vi "Automatic Assembly DB.vi"() -> ()   [LabVIEW 2021]
uses:
  Classes/Assembly/Assembly Run.lvclass
  Classes/Assembly/Database Entry/Database Entry.lvclass
  <vilib>/Utility/file.llb/Read Delimited Spreadsheet (string).vi
  SubVIs/PUT_region.vi
  SubVIs/component_tray_region.vi
  SubVIs/assembly_tray_region.vi
  Classes/Controller/I-O/I-O.lvclass
  Classes/Controller/Controller.lvclass
panel:
  in  "Abort assembly":bool
  in  "Do old-style single-module data-entry?":bool
  out "Status":string
  out "Stack names":T1
  out "Feet check":bool
  out "Assembly Type":string
  out "Assembly tray region":dbl
  out "Component tray region":dbl
  out "PUT Region":dbl
  # "Click the Run arrow to start.\nFill out pop-up prompts.\nSee Status for more info.\nAnswer ALL prompts until program stops running!"
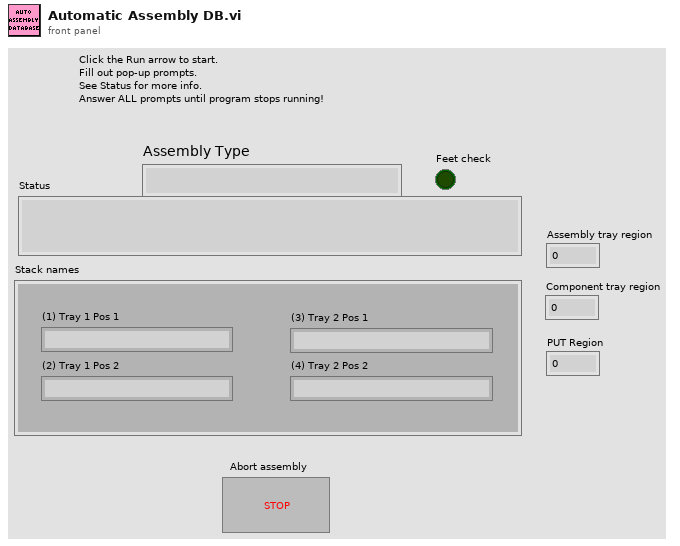
[diagram p1: front panel]
types:
  T1 = cluster{"(1) Tray 1 Pos 1":string, "(2) Tray 1 Pos 2":string, "(3) Tray 2 Pos 1":string, "(4) Tray 2 Pos 2":string}
  T2 = typedef "Controller.lvclass/Controllers.ctl" = cluster{"I-O.lvclass":refnum<class "I-O.lvclass">, "Gantry":refnum<k24>, "Dispenser":refnum<visa-resource-name>}
  T3 = typedef "File Paths.ctl" = cluster{"Glue Pattern Folder":path, "Carrier Tray Folder":path, "Pick Up Tool Fixture Folder":path, "Components Folder":path, "Bellows Tool Offset.txt":path, "Pick Up Tool Offset.txt":path, "Dispense Tip Offset.txt":path, "Log Files":path, "Gantry Assembly Map.txt":path, "Syringe and offset map.txt":path, "Controllers Folder":path, "Local dbase config":path}
  T4 = cluster{"Fixture ID":dbl, "Position":dbl, "Thickness":dbl}[]
  T5 = cluster{"Fixture ID":dbl, "Position":dbl, "Thickness":dbl}[][]
  T6 = cluster{"Fixture ID":dbl, "Position":dbl, "Thickness":dbl}
  T7 = typedef "I-O.lvclass/Pin Map.ctl" = cluster{"Region Valves":i32[], "Extra Valves":dbl[][][], "Tool Primary Valve":i32, "Tool Secondary Valve":i32, "Region Sensors":i32[], "Extra Sensors":dbl[][][], "Tool Primary Sensor":dbl, "Tool Secondary Sensor":dbl, "Compression Sensor":dbl, "5V":i32, "Dispenser Sensor":dbl, "Light Curtain":i32}
  T8 = cluster{"Stack names[0]":string, "Stack names[1]":string, "Stack names[2]":string, "Stack names[3]":string}
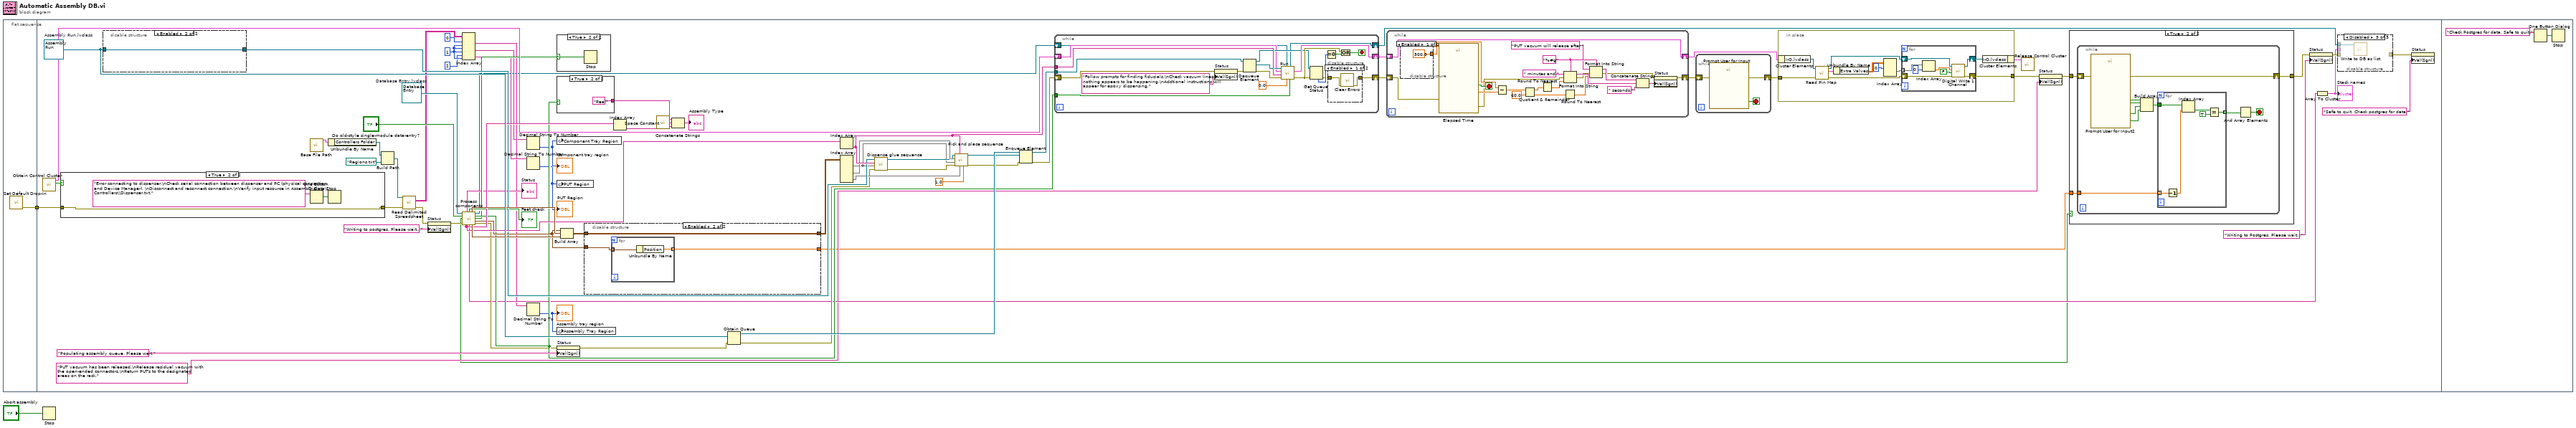
[diagram p0: block diagram]
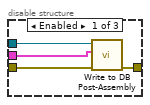
[diagram p3: hidden frame]
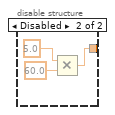
[diagram p5: hidden frame]
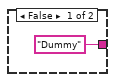
[diagram p7: hidden frame]
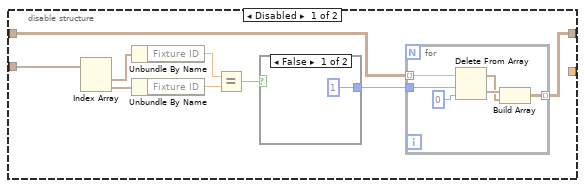
[diagram p9: hidden frame]
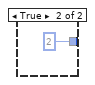
[diagram p10: hidden frame]
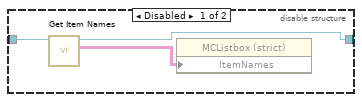
[diagram p11: hidden frame]
diagram:
  n1 = flat-sequence {
    tunnel: [w3] -> w2
    tunnel: w2 -> [w21]
    frame #0 {
      n2 = call "Set Default Drop-In.vi"() -> ("error out"=w3:errorcluster)  [unwired: 11 in]
    }
    frame #1 {
      w26 = 1 ("disabled index (col)")
      w49 = refnum<class "Database Entry.lvclass"> refnum  # Database Entry.lvclass
      w75 = refnum<class "Assembly Run.lvclass"> refnum  # Assembly Run.lvclass
      n3 = call "Obtain Control Cluster.vi"() -> ("Dispenser error?"=w38:bool, "Control Out"=w68:T2)  [unwired: 10 in]
      n4 = case shown="True" w38 {
        tunnel: w21 -> [w148 w149]
        tunnel: [w148 w149] -> w20
        frame False {
        }
        frame True {
          n5 = One Button Dialog(message="Error connecting to dispenser.\nCheck serial connection between dispenser and PC (physical connection and Device Manager). \nDisconnect and reconnect connection.\nVerify input resource in Assembly Data\\Controllers\\Dispenser.txt.") -> (true=w150:bool)  [unwired: 1 in]
          n6 = Stop(stop? (T)=w150) -> ()
        }
      }
      n7 = disable-structure shown="Enabled" {
        disable-tunnel: w75 -> [w179 w180]
        disable-tunnel: [w177 w180] -> w67
        frame Disabled {
          n8 = call "Get Item Names.vi"("Assembly Run in"=w179) -> ("Item names"=w178:string[][], "Assembly Run out"=w177:refnum<class "Assembly Run.lvclass">)  [unwired: 8 in, 1 out]
          n9 = property class="MCListbox (strict)"("ItemNames"=w178) -> ()  [unwired: 2 in, 2 out]
        }
        frame Enabled {
        }
      }
      n10 = call "Base File Path.vi"() -> ("Paths Out"=w37:T3)  [unwired: 11 in]
      n11 = Unbundle By Name(w37) -> ("Controllers Folder"=w35:path)
      n12 = Build Path(base path=w35, name or relative path=path "Regions.txt") -> (appended path=w36:path)
      n13 = call-poly <vilib>:"Read Delimited Spreadsheet.vi"("file path (dialog if empty)"=w36, "error in (no error)"=w20) -> ("all rows"=w24:string[][], "error out"=w22:errorcluster)  [unwired: 8 in, 4 out]
      n14 = property on="Status" class="Str"(error in=w22, "Val(Sgnl)"="Writing to postgres. Please wait..." ("Value (Signaling)")) -> (error out=w39:errorcluster)  [unwired: 1 in, 1 out]
      n15 = Index Array(array=w24, index (row) #1=0 ("index (row)"), index (col) #1=w26, index (row) #2=w26, index (col) #2=w26, index (row) #3=2 ("disabled index (row)"), index (col) #3=w26) -> (element #1=w29:string, element #2=w28:string, element #3=w30:string)
      n16 = call "Process components.vi"("Database Entry in"=w49, "Do single-module data entry?"="Do old-style single-module data-entry?", "error in (no error)"=w39) -> ("Status"=→"Status":string, "Feet check"=→"Feet check":bool, "PUT Settings"=w73:T4, "Database Entry out"=w5:refnum<class "Database Entry.lvclass">, "Is real run?"=w56:bool, "Module?"=w7:bool, "Aborted"=w46:bool, "Assembly Settings"=w69:T4, "Assembly Type"=w72:string[], "Stack names"=w48:string[], "Component Settings"=w74:T4, "error out"=w51:errorcluster)  [unwired: 1 in]
      n17 = Decimal String To Number(string=w28) -> (number=w33:i32)  [unwired: 2 in, 1 out]
      "Component tray region" <- w33
      n18 = Decimal String To Number(string=w30) -> (number=w31:i32)  [unwired: 2 in, 1 out]
      "PUT Region" <- w31
      n19 = Decimal String To Number(string=w29) -> (number=w32:i32)  [unwired: 2 in, 1 out]
      "Assembly tray region" <- w32
      n20 = case shown="True" w46 {
        selector: w46 -> [_ w154]
        frame False {
        }
        frame True {
          n21 = Stop(stop? (T)=w154) -> ()
        }
      }
      n22 = case shown="True" w56 {
        tunnel: ["Dummy" "Real"] -> w41
        frame False {
        }
        frame True {
        }
      }
      n23 = global write "component_tray_region.vi" "Component Tray Region"(w33) -> ()
      n24 = global write "PUT_region.vi" "PUT Region"(w31) -> ()
      n25 = global write "assembly_tray_region.vi" "Assembly Tray Region"(w32) -> ()
      n26 = property on="Status" class="Str"(error in=w51, "Val(Sgnl)"="Populating assembly queue. Please wait." ("Value (Signaling)")) -> (error out=w50:errorcluster)  [unwired: 1 in, 1 out]
      n27 = Build Array(w69, w73, w74) -> (w65:T5)
      n28 = disable-structure shown="Enabled" {
        disable-tunnel: w69 -> [w163 w173]
        disable-tunnel: [w162 w174] -> w66
        disable-tunnel: w65 -> [w161 w174]
        disable-tunnel: [_ w172] -> w6
        frame Disabled {
          n29 = Index Array(array=w163) -> (element #1=w160:T6, element #2=w159:T6)  [unwired: 2 in]
          n30 = Unbundle By Name(w160) -> ("Fixture ID"=w158:dbl)
          n31 = Unbundle By Name(w159) -> ("Fixture ID"=w157:dbl)
          n32 = Equal?(x=w158, y=w157) -> (x = y?=w156:bool)
          n33 = case shown="False" w156 {
            tunnel: [1 2] -> w155
            frame False {
            }
            frame True {
            }
          }
          n34 = for {
            tunnel: w161 -> [w171] mode=indexing
            tunnel: [w170] -> w162 mode=indexing
            tunnel: w155 -> [w166]
            n35 = Delete From Array(array=w171, length=w166, index=0) -> (deleted portion=w168:T4, array with subset deleted=w167:T4)
            n36 = Build Array(w168, w167) -> (w170:T5)
          }
        }
        frame Enabled {
          n37 = for {
            tunnel: w173 -> [w176] mode=indexing
            tunnel: [w175] -> w172 mode=indexing
            n38 = Unbundle By Name(w176) -> ("Position"=w175:dbl)
          }
        }
      }
      n39 = Index Array(array=w72) -> (element=w43:string)  [unwired: 1 in]
      n40 = call <vilib>:"Space Constant.vi"() -> ("String"=w42:string)
      n41 = Concatenate Strings(w41, w42, w43) -> (→"Assembly Type":string)
      n42 = Obtain Queue(element data type=w75, error in (no error)=w50) -> (queue out=w70:refnum<queue>, error out=w52:errorcluster)  [unwired: 3 in, 1 out]
      n43 = Index Array(array=w72) -> (element=w71:string)  [unwired: 1 in]
      n44 = Index Array(array=w66) -> (element #1=w58:T4, element #2=w64:T4, element #3=w63:T4)  [unwired: 6 in]
      n45 = call "Dispense glue sequence.vi"("error in (no error)"=w52, "Assembly Tray Settings Array"=w58, "Assembly Type"=w71, "Assembly Run in"=w67) -> ("error out"=w53:errorcluster, "Assembly Run out"=w59:refnum<class "Assembly Run.lvclass">)  [unwired: 6 in]
      n46 = call "Pick and place sequence.vi"("Numeric"=1.0, "Component Tray map"=w63, "Assembly Type"=w71, "error in (no error)"=w53, "Assembly Tray map"=w58, "PUT map"=w64, "Assembly Run in"=w59) -> ("error out"=w54:errorcluster, "Assembly Run out"=w62:refnum<class "Assembly Run.lvclass">)  [unwired: 3 in]
      n47 = Enqueue Element(queue=w70, element=w62, error in (no error)=w54) -> (queue out=w61:refnum<queue>, error out=w55:errorcluster)  [unwired: 1 in, 1 out]
      n48 = while {
        shift-right: [w200] -> w60
        shift-left: w68 -> [w184]
        tunnel: w71 -> [w199]
        tunnel: w61 -> [w198]
        tunnel: w56 -> [w194]
        shift-right: [w183] -> w18
        shift-left: w55 -> [w193]
        shift-right: [w181] -> w4
        shift-left: w5 -> [w182]
        stop <- w196 stop-if-true
        n49 = property on="Status" class="Str"(error in=w193, "Val(Sgnl)"="Follow prompts for finding fiducials.\nCheck vacuum lines if nothing appears to be happening.\nAddtional instructions will appear for epoxy dispensing." ("Value (Signaling)")) -> (error out=w185:errorcluster)  [unwired: 1 in, 1 out]
        n50 = Dequeue Element(queue=w198, error in (no error)=w185) -> (queue out=w192:refnum<queue>, element=w189:refnum<class "Assembly Run.lvclass">, error out=w188:errorcluster)  [unwired: 1 in, 1 out]
        n51 = call-dynamic "Run.vi"("Dispense?"=w194, "Pickup_Test_Number"=0.0, "Database Entry in"=w182, "error in (no error)"=w188, "Assembly Type"=w199, "Control In"=w184, "Assembly In"=w189) -> ("error out"=w197:errorcluster, "Control Out"=w200:T2, "Database Entry out"=w181:refnum<class "Database Entry.lvclass">)  [unwired: 1 in, 1 out]
        n52 = Get Queue Status(queue=w192, error in (no error)=w197) -> (error out=w190:errorcluster, # elements in queue=w191:i32)  [unwired: 1 in, 6 out]
        n53 = Equal To 0?(x=w191) -> (x = 0?=w195:bool)
        n54 = disable-structure shown="Enabled" {
          disable-tunnel: w190 -> [w202 w203]
          disable-tunnel: [w201 w203] -> w183
          frame Enabled {
            n55 = call <vilib>:"Clear Errors.vi"("error in (no error)"=w202) -> ("error out"=w201:errorcluster)  [unwired: 5 in, 1 out]
          }
          frame Disabled {
          }
        }
        n56 = Or(x=w197, y=w195) -> (x .or. y?=w196:bool)
      }
      n57 = while {
        shift-right: [w139] -> w78
        shift-left: w60 -> [w139]
        shift-right: [w122] -> w77
        shift-left: w18 -> [w126]
        stop <- w143 stop-if-true
        w133 = "%#g" ("format string")
        n58 = disable-structure shown="Enabled" {
          disable-tunnel: [300.0 ("Time Target (s)") w146] -> w142
          frame Enabled {
          }
          frame Disabled {
            n59 = Multiply(x=5.0 ("duration"), y=60.0) -> (x*y=w146:dbl)
          }
        }
        n60 = call "Elapsed Time"("Time Target (s)"=w142, "error in (no error)"=w126) -> ("Elapsed Time (s)"=w141:dbl, "Time has Elapsed"=w143:bool, "error out"=w125:errorcluster)  [unwired: 10 in, 5 out]
        n61 = Subtract(x=w142, y=w141) -> (x-y=w138:dbl)
        n62 = Quotient & Remainder(x=w138, y=60.0) -> (x-y*floor(x/y)=w136:dbl, floor(x/y)=w135:dbl)
        n63 = Round To Nearest(number=w136) -> (nearest integer value=w128:dbl)
        n64 = Format Into String(format string=w133, initial string=" minutes and ", error in=w125, w128) -> (resulting string=w134:string, error out=w124:errorcluster)
        n65 = Round To Nearest(number=w135) -> (nearest integer value=w127:dbl)
        n66 = Format Into String(format string=w133, initial string="PUT vacuum will release after ", error in=w124, w127) -> (resulting string=w130:string, error out=w123:errorcluster)
        n67 = Concatenate Strings(w130, w134, " seconds." ("string")) -> (w137:string)
        n68 = property on="Status" class="Str"(error in=w123, "Val(Sgnl)"=w137) -> (error out=w122:errorcluster)  [unwired: 1 in, 1 out]
      }
      n69 = while {
        shift-right: [w205] -> w76
        shift-left: w77 -> [w206]
        stop <- w204 stop-if-true
        n70 = call "Prompt User for Input"("error in (no error)"=w206) -> ("Release?"=w204:bool, "error out"=w205:errorcluster)  [unwired: 16 in, 1 out]
      }
      n71 = in-place {
        in-place-border: w76 -> [w106]
        in-place-border: [w104] -> w16
        n72 = in-place-cluster #1(w78) -> ("I-O.lvclass"=w108:refnum<class "I-O.lvclass">)
        n73 = call-dynamic "Read Pin Map.vi"("error in (no error)"=w106, "I-O in"=w108) -> ("error out"=w105:errorcluster, "Pin Map 2"=w113:T7, "I-O out"=w110:refnum<class "I-O.lvclass">)  [unwired: 7 in]
        n74 = Unbundle By Name(w113) -> ("Extra Valves"=w112:dbl[][][])
        n75 = Index Array(array=w112, index (dim 0)=0 ("index (page)")) -> (element=w111:dbl[][])  [unwired: 2 in]
        n76 = for {
          tunnel: w111 -> [w121] mode=indexing
          shift-right: [w119] -> w107
          shift-left: w110 -> [w120]
          shift-right: [w114] -> w104
          shift-left: w105 -> [w115]
          n77 = Index Array(array=w121, index=0) -> (element=w118:dbl)
          n78 = call-dynamic "Digital Write 1 Channel.vi"("error constant"=w115, "Value"=FALSE, "Channel"=w118, "I-O.lvclass"=w120) -> ("error IO"=w114:errorcluster, "I-O.lvclass 2"=w119:refnum<class "I-O.lvclass">)  [unwired: 6 in]
        }
        n79 = in-place-cluster #1("I-O.lvclass"=w107) -> (w15:T2)
      }
      n80 = call "Release Control Cluster.vi"("output cluster"=w15) -> ()  [unwired: 11 in]
      n81 = property on="Status" class="Str"(error in=w16, "Val(Sgnl)"="PUT vacuum has been released.\nRelease residual vacuum with the open-ended connectors.\nReturn PUTs to the designated areas on the rack." ("Value (Signaling)")) -> (error out=w14:errorcluster)  [unwired: 1 in, 1 out]
      n82 = case shown="True" w7 {
        tunnel: w14 -> [w79 w82]
        tunnel: [w79 w81] -> w13
        tunnel: w6 -> [_ w80]
        frame False {
        }
        frame True {
          n83 = while {
            shift-right: [w91] -> w81
            shift-left: w82 -> [w92]
            tunnel: w80 -> [w86]
            stop <- w84 stop-if-true
            n84 = call "Prompt User for Input2"("error in (no error)"=w92) -> ("Pos4"=w87:bool, "Pos3"=w88:bool, "Pos2"=w89:bool, "Pos1"=w90:bool, "error out"=w91:errorcluster)  [unwired: 13 in, 1 out]
            n85 = Build Array(w90, w89, w88, w87) -> (w85:bool[])
            n86 = for {
              tunnel: w86 -> [w98] mode=indexing
              tunnel: w85 -> [w97]
              tunnel: [w93] -> w83 mode=indexing
              n87 = Decrement(x=w98) -> (x-1=w96:dbl)
              n88 = Index Array(array=w97, index=w96) -> (element=w95:bool)
              n89 = Equal?(x=w95, y=TRUE) -> (x = y?=w93:bool)
            }
            n90 = And Array Elements(Boolean array=w83) -> (logical AND=w84:bool)
          }
        }
      }
      n91 = property on="Status" class="Str"(error in=w13, "Val(Sgnl)"="Writing to Postgres. Please wait...") -> (error out=w10:errorcluster)  [unwired: 1 in, 1 out]
      n92 = Array To Cluster(array=w48) -> (cluster=w9:T8)
      "Stack names" <- w9
      n93 = disable-structure shown="Disabled" {
        disable-tunnel: w4 -> [w102 _ w103]
        disable-tunnel: w9 -> [w101 _ _]
        disable-tunnel: w10 -> [w100 _ _]
        disable-tunnel: [w99 _ _] -> w12
        frame Enabled {
          n94 = call "Write to DB Post-Assembly.vi"("error in (no error)"=w100, "Stack names"=w101, "Database Entry in"=w102) -> ("error out"=w99:errorcluster)  [unwired: 7 in, 1 out]
        }
        frame Disabled {
        }
        frame Disabled {
          n95 = call "Write to DB as list.vi"("Database Entry in"=w103) -> ()  [unwired: 8 in, 3 out]
        }
      }
      n96 = property on="Status" class="Str"(error in=w12, "Val(Sgnl)"="Safe to quit. Check postgres for data.") -> ()  [unwired: 1 in, 2 out]
    }
    frame #2 {
      n97 = One Button Dialog(message="Check Postgres for data. Safe to quit.") -> (true=w208:bool)  [unwired: 1 in]
      n98 = Stop(stop? (T)=w208) -> ()
    }
  }
  n99 = Stop(stop? (T)="Abort assembly") -> ()
